vi "Close.vi"(8 "error in (no error)":errorcluster caption="错误输入（无错误）", 11 "34401A 输入":refnum<class "34401A.lvclass">) -> (0 "error out":errorcluster caption="错误输出", 3 "34401A 输出":refnum<class "34401A.lvclass">)   [LabVIEW 2020, in "34401A.lvlib" / "34401A.lvclass"]
uses:
  34401A.lvclass
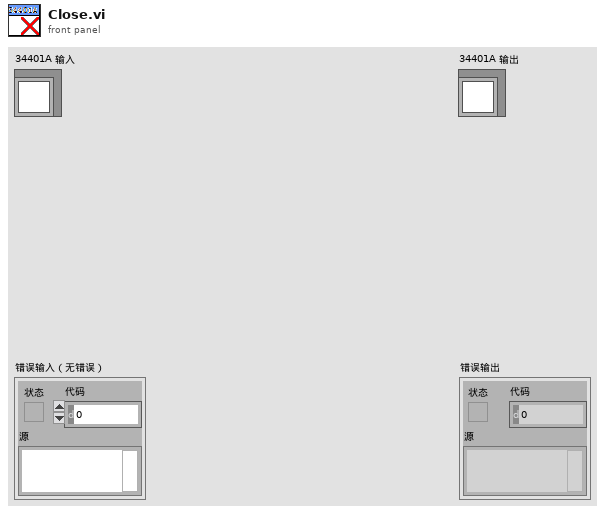
[diagram p1: front panel]
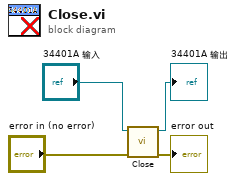
[diagram p0: block diagram]
diagram:
  n1 = call-parent "Close.vi"("error in (no error)"="error in (no error)", "数字多用表接口 输入"="34401A 输入") -> ("error out"=→"error out":errorcluster, "数字多用表接口 输出"=→"34401A 输出":refnum<class "34401A.lvclass">)  [unwired: 8 in]
